vi "Large array timing test.vi"() -> ()   [LabVIEW 2011]
uses:
  JSON Value/Get as JSON string.vi
  JSON Value/Set from JSON string.vi
  Variant JSON/Variant to JSON.vi
  Variant JSON/Get as Variant.vi
  JSON Value/Get Item by name array.vi
  JSON Value/JSON Value.lvclass
  Get Polymorphic/JSON GetSet.lvlib
  Variant JSON/Variant JSON.lvlib
panel:
  out "Variant out":variant
  out "to Variant":dbl format="%#_6p"
  out "from JSON":dbl format="%#_6p"
  out "To JSON":dbl format="%#_6p"
  out "Set Variant":dbl format="%#_6p"
  in  "Number":i32=10000
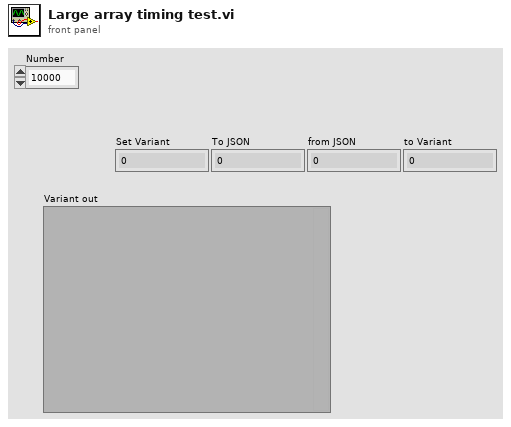
[diagram p1: front panel]
types:
  T1 = cluster{"B":cluster{"A":cluster{"Test":dbl[], "Test 2":dbl[], "Test 3":dbl[]}}}
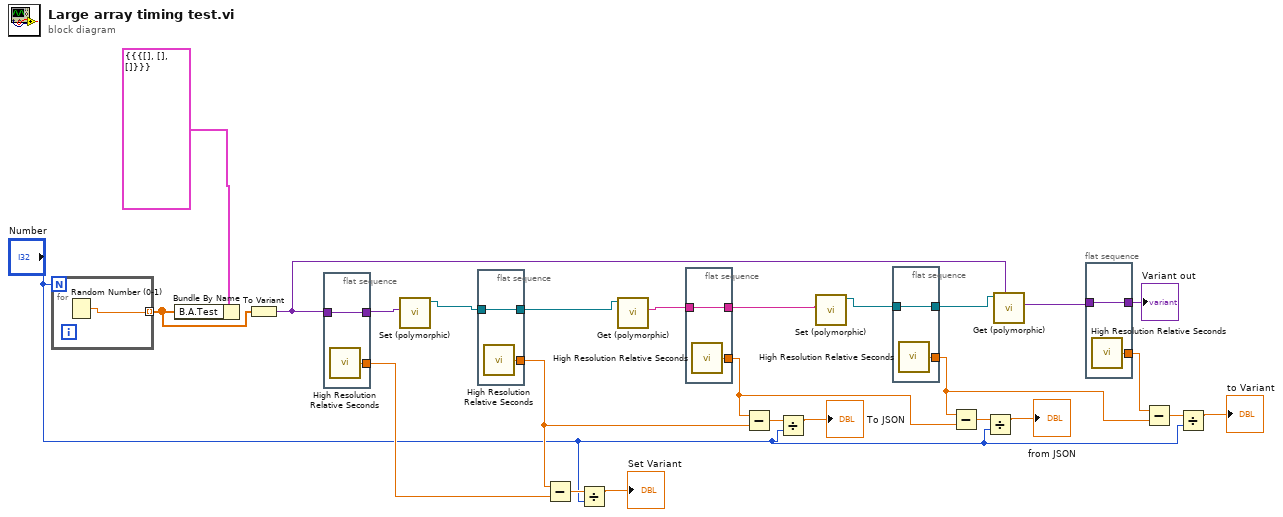
[diagram p0: block diagram]
diagram:
  n1 = for {
    N: "Number" -> [_]
    tunnel: [w27] -> w1 mode=indexing
    n2 = Random Number (0-1)() -> (number: 0 to 1=w27:dbl)
  }
  n3 = Bundle By Name(cluster=T1 {"B"={"A"={"Test"=[], "Test 2"=[], "Test 3"=[]}}}, "B.A.Test"=w1) -> ()  [unwired: 1 out]
  n4 = To Variant(anything=w1) -> (Variant=w10:variant)
  n5 = flat-sequence {
    tunnel: [w29] -> w26
    tunnel: w10 -> [w29]
    tunnel: [w28] -> w23
    frame #0 {
      n6 = call <vilib>:"High Resolution Relative Seconds.vi"() -> ("relative seconds"=w28:dbl)
    }
  }
  n7 = call-poly "Set (polymorphic).vi"("Variant"=w26) -> ("JSON Value out"=w25:refnum<class "JSON Value.lvclass">)  [unwired: 9 in, 1 out]
  n8 = flat-sequence {
    tunnel: [w31] -> w24
    tunnel: w25 -> [w31]
    tunnel: [w30] -> w17
    frame #0 {
      n9 = call <vilib>:"High Resolution Relative Seconds.vi"() -> ("relative seconds"=w30:dbl)
    }
  }
  n10 = Subtract(x=w17, y=w23) -> (x-y=w22:dbl)
  n11 = Divide(x=w22, y="Number") -> (x/y=→"Set Variant":dbl)
  n12 = call-poly "Get (polymorphic).vi"("JSON Value in"=w24) -> ("String"=w20:string)  [unwired: 9 in, 1 out]
  n13 = flat-sequence {
    tunnel: [w33] -> w16
    tunnel: w20 -> [w33]
    tunnel: [w32] -> w12
    frame #0 {
      n14 = call <vilib>:"High Resolution Relative Seconds.vi"() -> ("relative seconds"=w32:dbl)
    }
  }
  n15 = Subtract(x=w12, y=w17) -> (x-y=w18:dbl)
  n16 = Divide(x=w18, y="Number") -> (x/y=→"To JSON":dbl)
  n17 = call-poly "Set (polymorphic).vi"("JSON stream"=w16) -> ("JSON Value out"=w13:refnum<class "JSON Value.lvclass">)  [unwired: 8 in, 2 out]
  n18 = flat-sequence {
    tunnel: [w35] -> w11
    tunnel: w13 -> [w35]
    tunnel: [w34] -> w4
    frame #0 {
      n19 = call <vilib>:"High Resolution Relative Seconds.vi"() -> ("relative seconds"=w34:dbl)
    }
  }
  n20 = Subtract(x=w4, y=w12) -> (x-y=w15:dbl)
  n21 = Divide(x=w15, y="Number") -> (x/y=→"from JSON":dbl)
  n22 = call-poly "Get (polymorphic).vi"("Variant (Data Type)"=w10, "JSON in"=w11) -> ("Variant out"=w6:variant)  [unwired: 7 in, 2 out]
  n23 = flat-sequence {
    tunnel: [w37] -> w3
    tunnel: w6 -> [w37]
    tunnel: [w36] -> w7
    frame #0 {
      n24 = call <vilib>:"High Resolution Relative Seconds.vi"() -> ("relative seconds"=w36:dbl)
    }
  }
  n25 = Subtract(x=w7, y=w4) -> (x-y=w8:dbl)
  n26 = Divide(x=w8, y="Number") -> (x/y=→"to Variant":dbl)
  "Variant out" <- w3
